vi "MSScript_Calc_mathieu_beta.vi"(5 "Ion trap":cluster{"R0":ext, "Z0":ext}, 6 "Value Error?":bool[](array[boolean]), 8 "ArrayVariable in":ext[](array[numeric]), 9 "Param Items":i32) -> (0 "ArrayVariable out":ext[](array[numeric]), 2 "CmdError?":bool)   [LabVIEW 2018, in "MSScript.lvclass"]
uses:
  MSScript.lvclass
  PublicSubVI/Ctl/MathieuEqParam.ctl
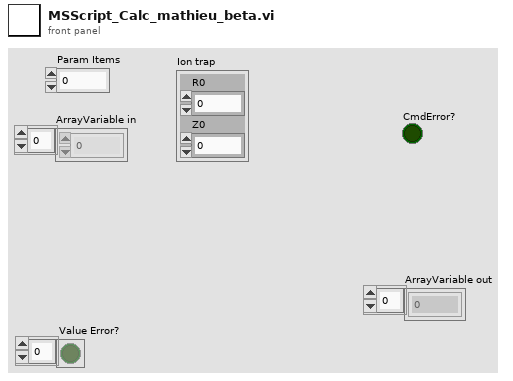
[diagram p1: front panel]
types:
  T1 = typedef "MathieuEqParam.ctl" = cluster{"mz(Th)":ext, "Amp(V)":ext, "Freq(Hz)":ext, "Beta":ext, "r_0 (mm)":ext, "z_0 (mm)":ext}
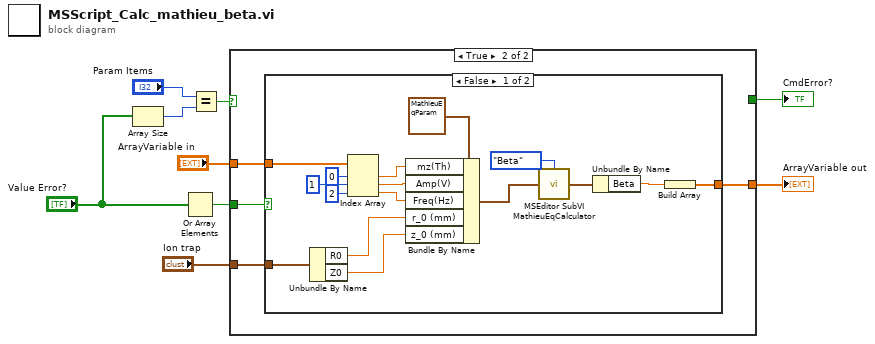
[diagram p0: block diagram]
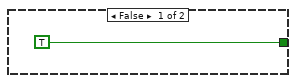
[diagram p2: hidden frame]
diagram:
  n1 = Array Size(array="Value Error?") -> (size(s)=w5:i32)
  n2 = Or Array Elements(Boolean array="Value Error?") -> (logical OR=w7:bool)
  n3 = Equal?(x="Param Items", y=w5) -> (x = y?=w3:bool)
  n4 = case shown="True" w3 {
    tunnel: [TRUE _] -> w2
    tunnel: w7 -> [_ w13]
    tunnel: "ArrayVariable in" -> [_ w14]
    tunnel: [_ w12] -> w9
    tunnel: "Ion trap" -> [_ w11]
    frame False {
    }
    frame True {
      n5 = case shown="False" w13 {
        tunnel: w14 -> [w28 _]
        tunnel: [w27 _] -> w12
        tunnel: w11 -> [w17 _]
        frame False {
          n6 = Unbundle By Name(w17) -> ("R0"=w16:ext, "Z0"=w15:ext)
          n7 = Index Array(array=w28, index #1=0 ("index"), index #2=1 ("index"), index #3=2 ("index")) -> (element #1=w21:ext, element #2=w20:ext, element #3=w19:ext)
          n8 = Bundle By Name(cluster=T1 {"mz(Th)"=0.0, "Amp(V)"=330.0, "Freq(Hz)"=0.0, "Beta"=1.0, "r_0 (mm)"=10.0, "z_0 (mm)"=7.07} ("Parametres 2"), "mz(Th)"=w21, "Amp(V)"=w20, "Freq(Hz)"=w19, "r_0 (mm)"=w16, "z_0 (mm)"=w15) -> (w24:T1)
          n9 = call "MSEditor SubVI MathieuEqCalculator.vi"("Target (Freq)"=enum16{"m/z", "Volt", "Freq", "Beta"}."Beta", "Parametres in"=w24) -> ("Parametres out"=w23:T1)  [unwired: 2 in]
          n10 = Unbundle By Name(w23) -> ("Beta"=w18:ext)
          n11 = Build Array(w18) -> (w27:ext[])
        }
        frame True {
        }
      }
    }
  }
  "ArrayVariable out" <- w9
  "CmdError?" <- w2
